vi "test Compile RaF Communication.vi"(8 "error in (no error)":errorcluster, 11 "TestCase in":refnum<class "Routing and Faulting Compile Unit Tests.lvclass">) -> (0 "error out":errorcluster, 3 "TestCase out":refnum<class "Routing and Faulting Compile Unit Tests.lvclass">)   [LabVIEW 2017, in "Routing and Faulting Compile Unit Tests.lvclass"]
uses:
  Routing and Faulting Compile Unit Tests.lvclass
  Shared/Communication Configuration.ctl
  Shared/Compiled.Settings.ctl
  Shared/Routing and Faulting Configuration.ctl
  Shared/Routing Channel Configuration.ctl
  Shared/Value-Connections Map.ctl
  Shared/Connection.ctl
  Shared/Alias Mapping.ctl
  Shared/FIFO Indices.ctl
  Routing and Faulting Compile Unit Tests.lvclass/Routing and Faulting Compile Unit Tests.ctl
  Shared/Routing and Faulting Shared.lvlib
  Scripting/Switch Scripting.lvlib
  System Explorer/Routing and Faulting System Explorer.lvlib
panel:
  out "Communication Configuration":T1
  in  "Save?":bool
  out "Output Filename":string
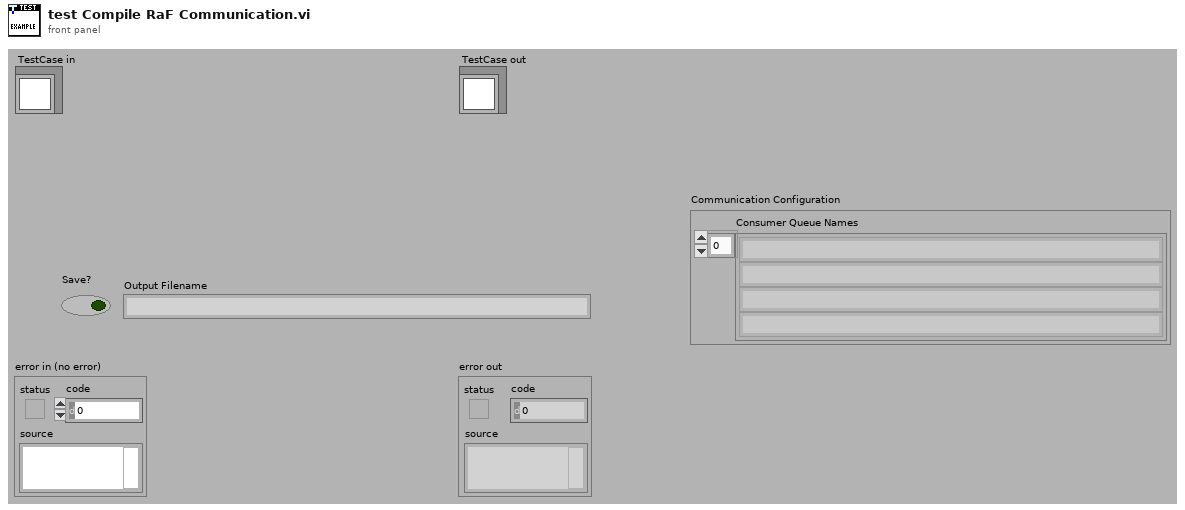
[diagram p1: front panel]
types:
  T1 = typedef "Routing and Faulting Shared.lvlib/Communication Configuration.ctl" = cluster{"Consumer Queue Names":string[]}
  T2 = typedef "Routing and Faulting Shared.lvlib/Compiled.Settings.ctl" = cluster{"Custom Device Name":string, "Communication Configuration":T1, "Routing and Faulting Configuration":T3, "Status Channels FIFO Indices":T8}
  T3 = typedef "Routing and Faulting Shared.lvlib/Routing and Faulting Configuration.ctl" = cluster{"Routing Channel Configurations":T4[], "Alias Mappings":T7[]}
  T4 = typedef "Routing and Faulting Shared.lvlib/Routing Channel Configuration.ctl" = cluster{"Channel Name":string, "Initial Value":dbl, "FIFO Index":i32, "Value-Connections Map":T5}
  T5 = typedef "Routing and Faulting Shared.lvlib/Value-Connections Map.ctl" = cluster{"State Value Array":i32[], "Connection List Array":cluster{"Connection List":T6[]}[]}
  T6 = typedef "Routing and Faulting Shared.lvlib/Connection.ctl" = cluster{"Source":string, "Destination":string}
  T7 = typedef "Routing and Faulting Shared.lvlib/Alias Mapping.ctl" = cluster{"Endpoint":string, "Alias":string}
  T8 = typedef "Routing and Faulting Shared.lvlib/FIFO Indices.ctl" = cluster{"Status Channel":i32, "Heartbeat Channel":i32}
  T9 = typedef "Custom Device API.lvlib/Custom Device Item Ref.ctl" = u64
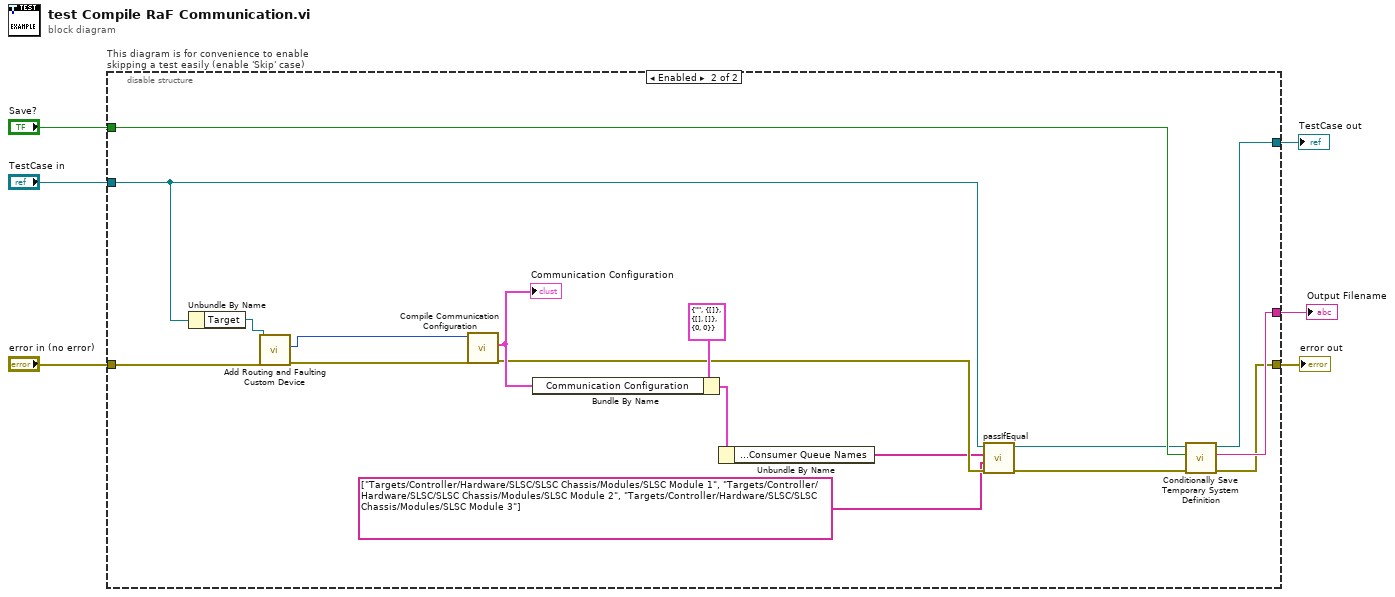
[diagram p0: block diagram]
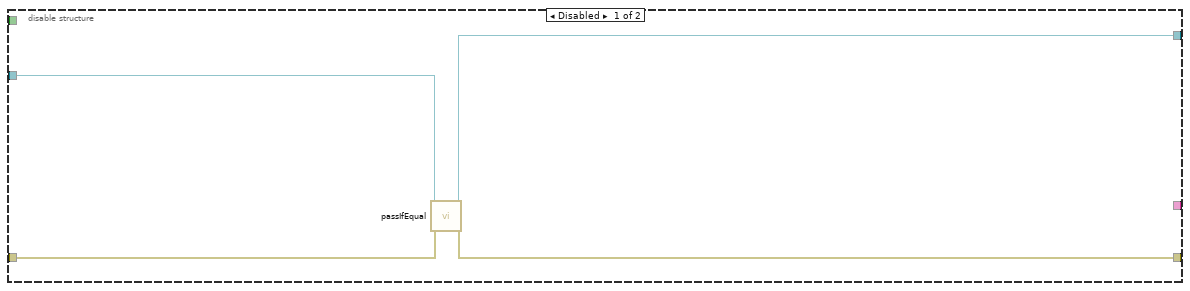
[diagram p2: hidden frame]
diagram:
  n1 = disable-structure "This diagram is for convenience to enable skipping a test easily (enable 'Skip' case)" shown="Enabled" {
    disable-tunnel: "TestCase in" -> [w10 w22]
    disable-tunnel: [w9 w24] -> w3
    disable-tunnel: [w8 w20] -> w5
    disable-tunnel: "error in (no error)" -> [w7 w26]
    disable-tunnel: "Save?" -> [_ w25]
    disable-tunnel: [_ w23] -> w1
    frame Disabled {
      n2 = call-dynamic "passIfEqual.vi"("error in (no error)"=w7, "TestCase in"=w10) -> ("error out"=w8:errorcluster, "TestCase out"=w9:refnum<class "Routing and Faulting Compile Unit Tests.lvclass">)  [unwired: 8 in]
    }
    frame Enabled {
      n3 = Unbundle By Name(w22) -> ("Target"=w27:refnum<k24>)
      n4 = call "Add Routing and Faulting Custom Device.vi"("error in (no error)"=w26, "Target in"=w27) -> ("error out"=w18:errorcluster, "Routing and Faulting Custom Device Ref"=w15:T9)  [unwired: 7 in, 1 out]
      n5 = call "Compile Communication Configuration.vi"("error in (no error)"=w18, "Device Ref in"=w15) -> ("error out"=w14:errorcluster, "Communication Configuration"=w16:T1)  [unwired: 7 in, 1 out]
      "Communication Configuration" <- w16
      n6 = Bundle By Name(cluster=T2 {"Custom Device Name"="", "Communication Configuration"={"Consumer Queue Names"=[]}, "Routing and Faulting Configuration"={"Routing Channel Configurations"=[], "Alias Mappings"=[]}, "Status Channels FIFO Indices"={"Status Channel"=0, "Heartbeat Channel"=0}} ("Compiled.Settings.ctl"), "Communication Configuration"=w16) -> (w13:T2)
      n7 = Unbundle By Name(w13) -> ("Communication Configuration.Consumer Queue Names"=w12:string[])
      n8 = call-dynamic "passIfEqual.vi"("error in (no error)"=w14, "y"=string[] ["Targets/Controller/Hardware/SLSC/SLSC Chassis/Modules/SLSC Module 1", "Targets/Controller/Hardware/SLSC/SLSC Chassis/Modules/SLSC Module 2", "Targets/Controller/Hardware/SLSC/SLSC Chassis/Modules/SLSC Module 3"] ("Consumer Queue Names"), "x"=w12, "TestCase in"=w22) -> ("error out"=w19:errorcluster, "TestCase out"=w21:refnum<class "Routing and Faulting Compile Unit Tests.lvclass">)  [unwired: 6 in]
      n9 = call "Conditionally Save Temporary System Definition.vi"("error in (no error)"=w19, "Save?"=w25, "TestCase in"=w21) -> ("error out"=w20:errorcluster, "filename"=w23:string, "TestCase out"=w24:refnum<class "Routing and Faulting Compile Unit Tests.lvclass">)  [unwired: 6 in]
    }
  }
  "error out" <- w5
  "TestCase out" <- w3
  "Output Filename" <- w1
